vi "output_line_offset_fixed x_3D.vi"(7 "# of samples":i32=10000, 9 "Offset / V":cluster{"X":dbl, "Y":dbl, "Z":dbl}={"X"=0.1, "Y"=0.4, "Z"=0.5}) -> (1 "Falling Slope":dbl[][](graph), 2 "Rising slope":dbl[][](graph))   [LabVIEW 2018]
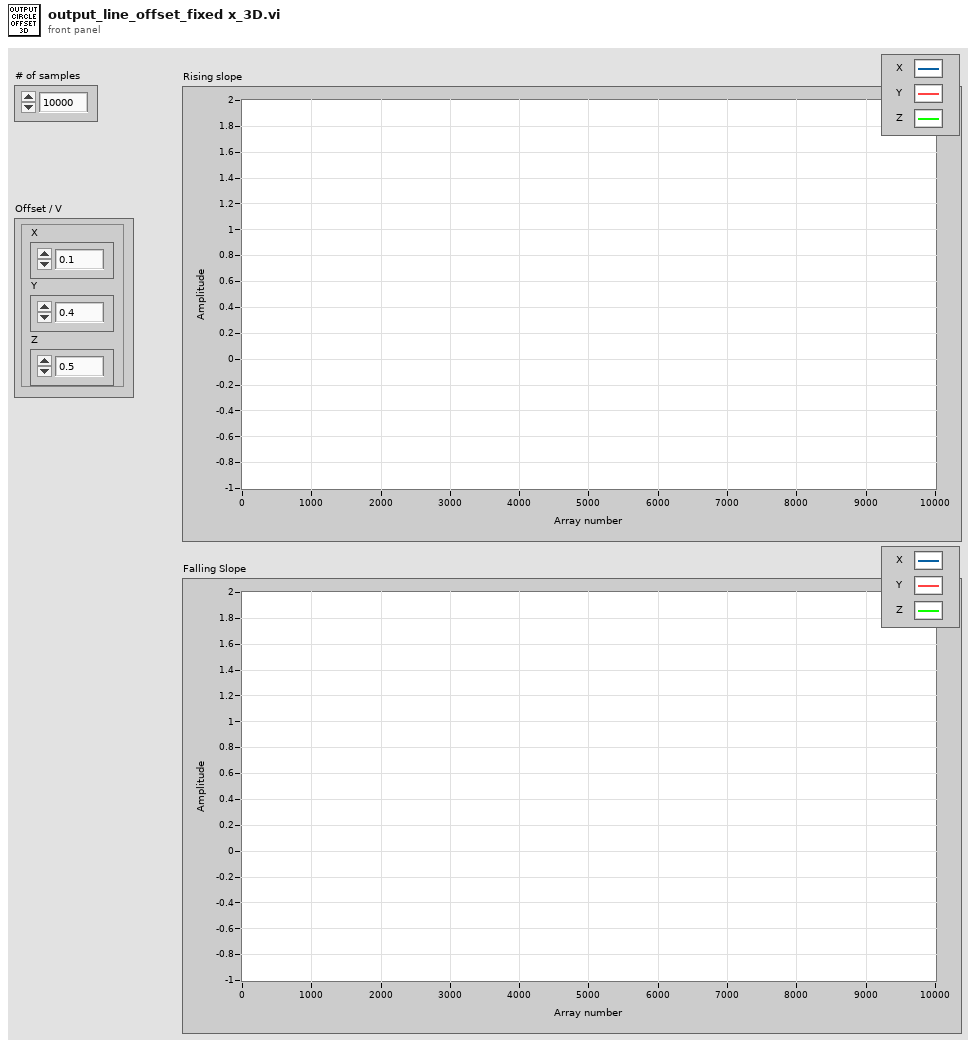
[diagram p1: front panel]
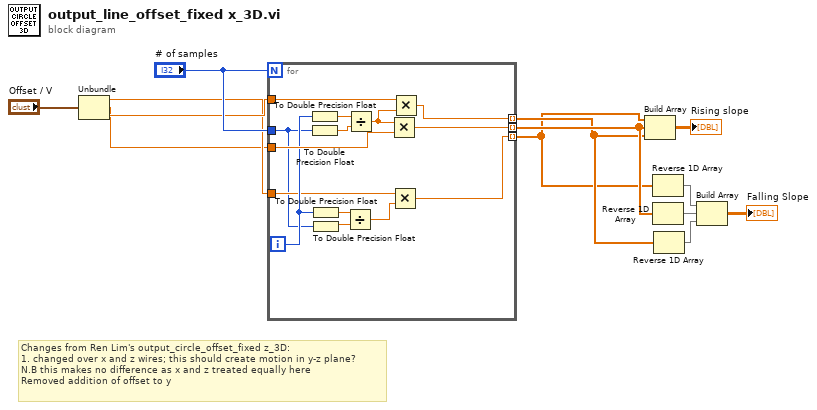
[diagram p0: block diagram]
diagram:
  # "Changes from Ren Lim's output_circle_offset_fixed z_3D:\n1. changed over x and z wires; this should create motion in y-z plane?\nN.B this makes no difference as x and z treated equally here\nRemoved addition of offset to y"
  n1 = Unbundle("Offset / V") -> ("X"=w4:dbl, "Y"=w1:dbl, "Z"=w5:dbl)
  n2 = for {
    N: "# of samples" -> [_]
    tunnel: "# of samples" -> [w17]
    tunnel: w1 -> [w25]
    tunnel: [w24] -> w11 mode=indexing
    tunnel: [w14] -> w3 mode=indexing
    tunnel: w5 -> [w22]
    tunnel: w4 -> [w18]
    tunnel: [w16] -> w2 mode=indexing
    i -> [w21]
    n3 = To Double Precision Float(number=w21) -> (double precision float=w27:dbl)
    n4 = To Double Precision Float(number=w17) -> (double precision float=w26:dbl)
    n5 = To Double Precision Float(number=w21) -> (double precision float=w20:dbl)
    n6 = To Double Precision Float(number=w17) -> (double precision float=w15:dbl)
    n7 = Divide(x=w20, y=w15) -> (x/y=w19:dbl)
    n8 = Divide(x=w27, y=w26) -> (x/y=w23:dbl)
    n9 = Multiply(x=w23, y=w25) -> (x*y=w24:dbl)
    n10 = Multiply(x=w18, y=w19) -> (x*y=w16:dbl)
    n11 = Multiply(x=w22, y=w23) -> (x*y=w14:dbl)
  }
  n12 = Build Array(w2, w11, w3) -> (→"Rising slope":dbl[][])
  n13 = Reverse 1D Array(array=w2) -> (reversed array=w8:dbl[])
  n14 = Reverse 1D Array(array=w11) -> (reversed array=w10:dbl[])
  n15 = Reverse 1D Array(array=w3) -> (reversed array=w6:dbl[])
  n16 = Build Array(w8, w10, w6) -> (→"Falling Slope":dbl[][])
